vi "LVClass_CorrectionDataManager Read CorrectionDataManager.vi"(8 "error in (no error)":errorcluster, 11 "CorrectionDataManager in":refnum<class "CorrectionDataManager.lvclass">) -> (0 "error out":errorcluster, 2 "CorrectionDataManager":T1, 3 "CorrectionDataManager out":refnum<class "CorrectionDataManager.lvclass">)   [LabVIEW 2020, in "CorrectionDataManager.lvclass"]
uses:
  CorrectionDataManager.lvclass
  ClassID.ctl
  CorrectionDataManager.lvclass/CorrectionDataManager.ctl
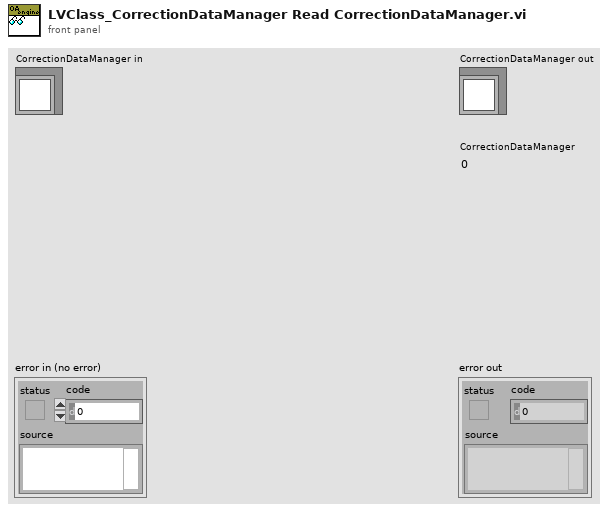
[diagram p1: front panel]
types:
  T1 = typedef "ClassID.ctl" = i64
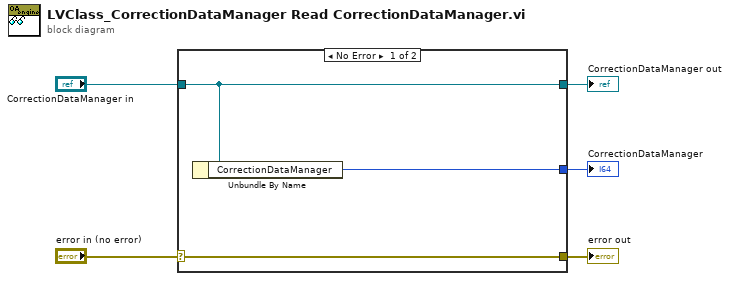
[diagram p0: block diagram]
diagram:
  n1 = case shown="No Error" "error in (no error)" {
    selector: "error in (no error)" -> [w8 w9]
    tunnel: [w8 w9] -> w4
    tunnel: [w7 w10] -> w2
    tunnel: "CorrectionDataManager in" -> [w7 w10]
    tunnel: [w6 _] -> w1
    frame No Error {
      n2 = Unbundle By Name(w7) -> ("CorrectionDataManager"=w6:T1)
    }
    frame Error {
    }
  }
  "error out" <- w4
  "CorrectionDataManager out" <- w2
  "CorrectionDataManager" <- w1
